vi "Stop Acquisition.vi"(8 "error in":errorcluster, 11 "HW Refnum":string) -> (0 "error out":errorcluster)   [LabVIEW 2020, in "Acquisition.lvlib"]
doc: "Stops the acquisition.\n_____\nBased on DQMH Project Template 7.0.1.1316."
uses:
  Acquisition.lvlib
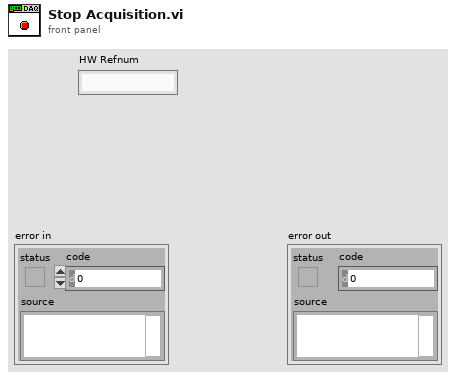
[diagram p1: front panel]
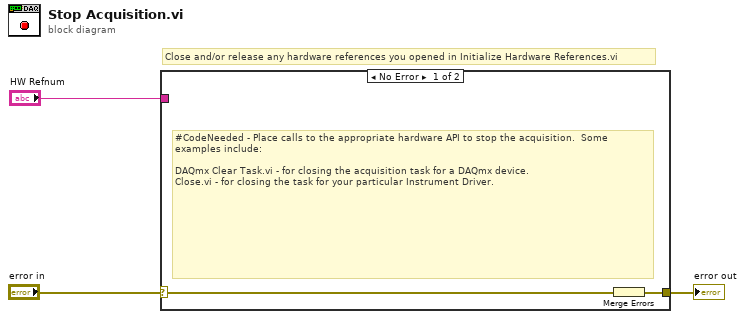
[diagram p0: block diagram]
diagram:
  # "Close and/or release any hardware references you opened in Initialize Hardware References.vi"
  n1 = case shown="No Error" "error in" {
    selector: "error in" -> [w4 w6]
    tunnel: [w5 w6] -> w2
    tunnel: "HW Refnum" -> [_ _]
    frame No Error {
      # "#CodeNeeded - Place calls to the appropriate hardware API to stop the acquisition.  Some examples include:\n\nDAQmx Clear Task.vi - for closing the acquisition task for a DAQmx device.\nClose.vi - for closing the task for your particular Instrument Driver."
      n2 = Merge Errors(w4) -> (w5:errorcluster)
    }
    frame Error {
    }
  }
  "error out" <- w2
